vi "Untitled 1.vi"() -> ()   [LabVIEW 2024]
panel:
  out "Waveform Chart":dbl(graph)
  in  "stop":bool
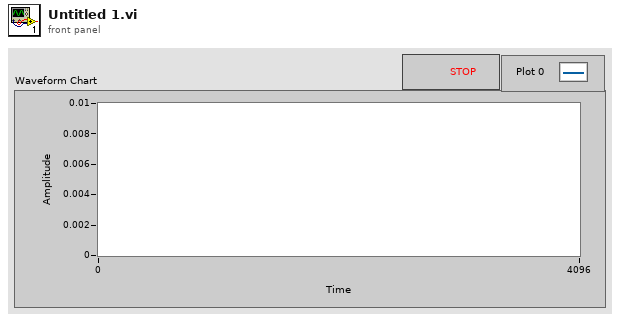
[diagram p1: front panel]
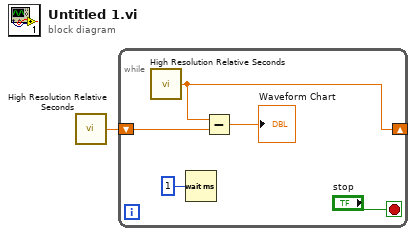
[diagram p0: block diagram]
diagram:
  n1 = call <vilib>:"High Resolution Relative Seconds.vi"() -> ("relative seconds"=w1:dbl)
  n2 = while {
    shift-right: [w4] -> _
    shift-left: w1 -> [w3]
    stop <- "stop" stop-if-true
    n3 = call <vilib>:"High Resolution Relative Seconds.vi"() -> ("relative seconds"=w4:dbl)
    n4 = Wait (ms)(milliseconds to wait=u32 1) -> ()  [unwired: 1 out]
    n5 = Subtract(x=w4, y=w3) -> (x-y=→"Waveform Chart":dbl)
  }
